vi "Assigning VICI Letter.vi"() -> ()   [LabVIEW 2018, in "VICI M6 M50 Party Mode.lvlib"]
uses:
  VICI M6 M50 Party Mode.lvlib
  <vilib>/Instr/_visa.llb/VISA Configure Serial Port (Instr).vi
panel:
  out "Bytes at Port 5":u32
  out "read buffer 8":string
  out "String 2":string
  out "Bytes at Port 7":u32
  out "read buffer 3":string
  out "Already Labeled":bool
  out "error out":errorcluster
  out "String":string
  out "Bytes at Port 6":u32
  out "read buffer 2":string
  out "output array":string[](array[string])
  out "Bytes at Port 4":u32
  out "read buffer 7":string
  out "Bytes at Port 3":u32
  out "read buffer 6":string
  in  "VISA resource name":refnum<visa-resource-name>
  in  "error in (no error)":errorcluster
  out "read buffer 5":string
  out "Bytes at Port":u32
  out "read buffer":string
  out "Bytes at Port 2":u32
  in  "Pump Letter (single, case sensitive letter of number)":string
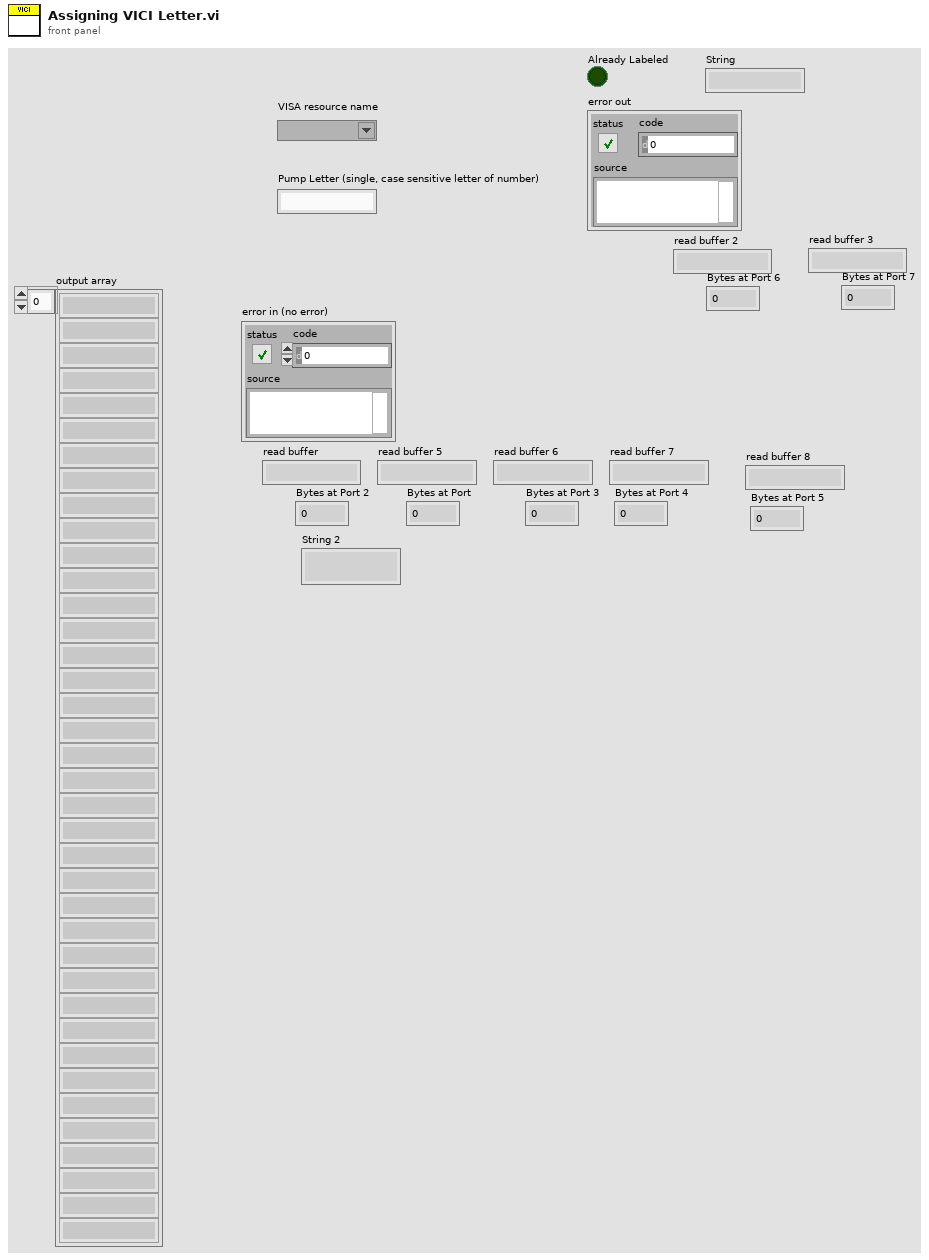
[diagram p1: front panel]
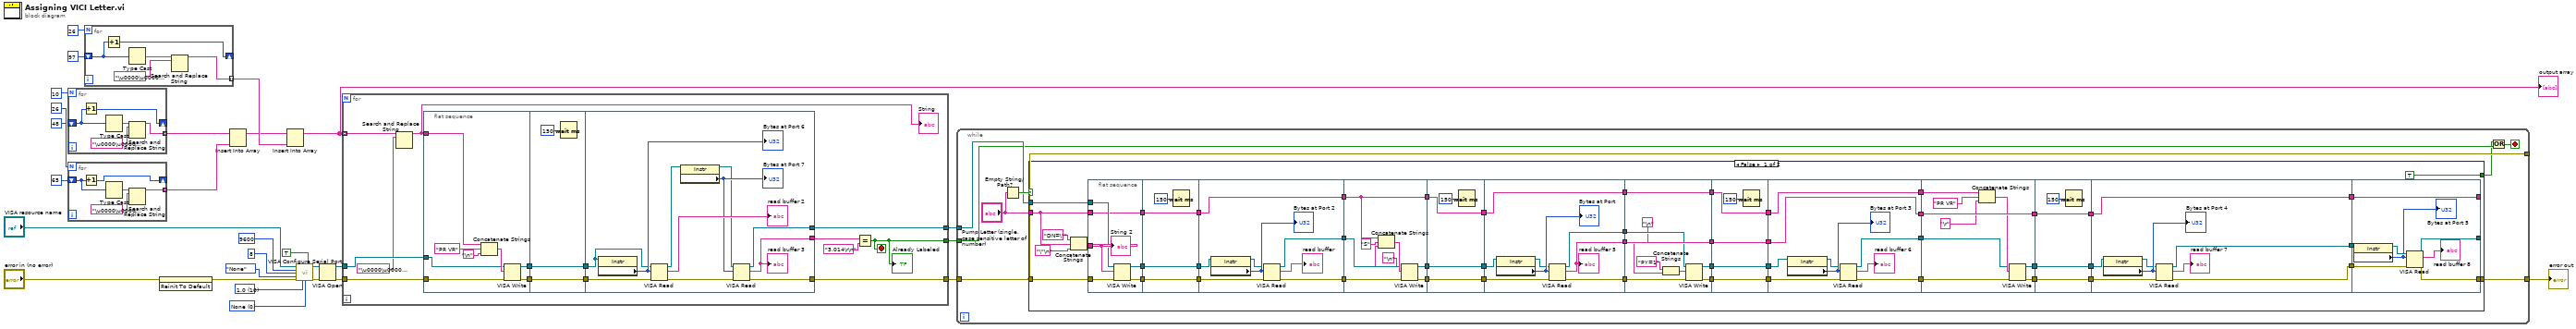
[diagram p0: block diagram]
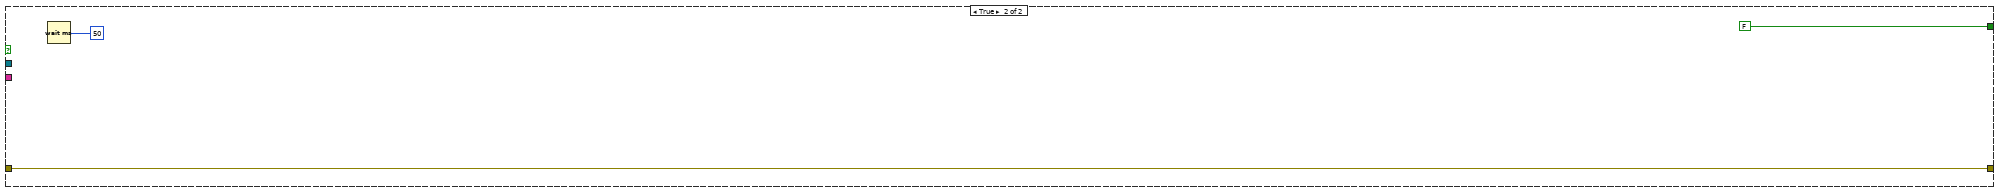
[diagram p2: hidden frame]
diagram:
  w23 = u16 0 items=["None", "XON/XOFF", "RTS/CTS", "XON/XOFF & RTS/CTS", "DTR/DSR", "XON/XOFF & DTR/DSR"] ("flow control (0:none)")
  w24 = u16 10 items=["1.0"=10, "1.5"=15, "2.0"=20] ("stop bits (10: 1 bit)")
  n1 = for {
    N: 10 -> [_]
    shift-right: [w33] -> _
    shift-left: 48 -> [w32]
    tunnel: [w29] -> w8 mode=indexing
    n2 = Increment(x=w32) -> (x+1=w33:i32)
    n3 = Type Cast(x=w32) -> (*(type *) &x=w30:string)  [unwired: 1 in]
    n4 = Search and Replace String(input string=w30, search string="\u0000\u0000\u0000") -> (result string=w29:string)  [unwired: 6 in, 3 out]
  }
  n5 = for {
    N: 26 -> [_]
    shift-right: [w38] -> _
    shift-left: 65 -> [w37]
    tunnel: [w34] -> w9 mode=indexing
    n6 = Increment(x=w37) -> (x+1=w38:i32)
    n7 = Type Cast(x=w37) -> (*(type *) &x=w35:string)  [unwired: 1 in]
    n8 = Search and Replace String(input string=w35, search string="\u0000\u0000\u0000") -> (result string=w34:string)  [unwired: 6 in, 3 out]
  }
  n9 = for {
    N: 26 -> [_]
    shift-right: [w43] -> _
    shift-left: 97 -> [w42]
    tunnel: [w39] -> w11 mode=indexing
    n10 = Increment(x=w42) -> (x+1=w43:i32)
    n11 = Type Cast(x=w42) -> (*(type *) &x=w40:string)  [unwired: 1 in]
    n12 = Search and Replace String(input string=w40, search string="\u0000\u0000\u0000") -> (result string=w39:string)  [unwired: 6 in, 3 out]
  }
  n13 = invoke on="Pump Letter (single, case sensitive letter of number)" class="Str" method="Reinit To Default"(error in="error in (no error)") -> (error out=w19:errorcluster)  [unwired: 2 in, 2 out]
  n14 = Insert Into Array(array=w8, new element=w9) -> (w10:string[])  [unwired: 1 in]
  n15 = Insert Into Array(array=w10, new element=w11) -> (w1:string[])  [unwired: 1 in]
  "output array" <- w1
  n16 = call-poly "VISA Configure Serial Port"("VISA resource name"="VISA resource name", "Enable Termination\nChar (T)"=TRUE ("Enable Termination\nChar (T)"), "baud rate (9600)"=u32 9600, "data bits (8)"=u16 8, "parity (0:none)"=enum16{"None", "Odd", "Even", "Mark", "Space"}."None", "error in (no error)"=w19, "stop bits (10: 1 bit)"=w24, "flow control (0:none)"=w23) -> ("VISA resource name out"=w21:refnum<visa-resource-name>, "error out"=w22:errorcluster)  [unwired: 6 in]
  n17 = VISA Open(error in (no error)=w22, VISA resource name=w21) -> (VISA resource name=w16:refnum<visa-resource-name>, error out=w17:errorcluster)  [unwired: 3 in]
  n18 = for {
    tunnel: w1 -> [w48] mode=indexing
    tunnel: w17 -> [w53]
    tunnel: w16 -> [w52]
    tunnel: [w50] -> w13
    tunnel: [w49] -> w14
    tunnel: [w44] -> w12
    stop <- w44 stop-if-true
    n19 = Search and Replace String(input string=w48, search string="\u0000\u0000\u0000") -> (result string=w47:string)  [unwired: 6 in, 3 out]
    "String" <- w47
    n20 = flat-sequence {
      tunnel: w47 -> [w64]
      tunnel: [w63] -> w56
      tunnel: [w62] -> w55
      tunnel: w53 -> [w61]
      tunnel: w52 -> [w60]
      tunnel: [w67] -> w57
      tunnel: w56 -> [w67]
      tunnel: w55 -> [w66]
      tunnel: [w66] -> w54
      tunnel: w57 -> [w78]
      tunnel: w54 -> [w77]
      tunnel: [w72] -> w50
      tunnel: [w74] -> w49
      tunnel: [w69] -> w45
      frame #0 {
        n21 = Concatenate Strings(w64, "PR VR" ("string"), "\n") -> (w65:string)
        n22 = VISA Write(VISA resource name=w60, write buffer=w65, error in (no error)=w61) -> (VISA resource name out=w63:refnum<visa-resource-name>, error out=w62:errorcluster)  [unwired: 1 out]
      }
      frame #1 {
        n23 = Wait (ms)(milliseconds to wait=u32 150) -> ()  [unwired: 1 out]
      }
      frame #2 {
        n24 = property class="Instr"(reference=w78) -> ("Serial Settings:Number of Bytes at Serial Port"=w79:u32)  [unwired: 1 in, 2 out]
        "Bytes at Port 6" <- w79
        n25 = VISA Read(VISA resource name=w78, byte count=w79, error in (no error)=w77) -> (VISA resource name out=w71:refnum<visa-resource-name>, read buffer=→"read buffer 2":string, error out=w73:errorcluster)  [unwired: 1 out]
        n26 = property class="Instr"(reference=w71) -> (reference out=w70:refnum<visa-resource-name>, "Serial Settings:Number of Bytes at Serial Port"=w75:u32)  [unwired: 1 in, 1 out]
        "Bytes at Port 7" <- w75
        n27 = VISA Read(VISA resource name=w70, byte count=w75, error in (no error)=w73) -> (VISA resource name out=w74:refnum<visa-resource-name>, read buffer=w69:string, error out=w72:errorcluster)  [unwired: 1 out]
        "read buffer 3" <- w69
      }
    }
    n28 = Equal?(x=w45, y="3.014\r\n") -> (x = y?=w44:bool)
    "Already Labeled" <- w44
  }
  n29 = while {
    tunnel: [w84] -> _
    tunnel: w14 -> [w85]
    tunnel: w13 -> [w84]
    tunnel: [w83] -> w15
    tunnel: w12 -> [w82]
    stop <- w80 stop-if-true
    n30 = Empty String/Path?(string/path="Pump Letter (single, case sensitive letter of number)") -> (empty?=w87:bool)
    n31 = case shown="False" w87 {
      tunnel: "Pump Letter (single, case sensitive letter of number)" -> [w117 _]
      tunnel: w84 -> [w122 w226]
      tunnel: [TRUE FALSE] -> w81
      tunnel: w85 -> [w121 _]
      tunnel: [w120 w226] -> w83
      frame False {
        n32 = Concatenate Strings("DN=\"" ("string"), w117, "\"\n" ("string")) -> (w116:string)
        n33 = flat-sequence {
          tunnel: [w140] -> w135
          tunnel: [w139] -> w134
          tunnel: w122 -> [w141]
          tunnel: w117 -> [w136]
          tunnel: w121 -> [w138]
          tunnel: w116 -> [w137]
          tunnel: [w136] -> w113
          tunnel: [w143] -> w133
          tunnel: w135 -> [w143]
          tunnel: w134 -> [w144]
          tunnel: [w144] -> w132
          tunnel: [w142] -> w114
          tunnel: w113 -> [w142]
          tunnel: w133 -> [w149]
          tunnel: w132 -> [w153]
          tunnel: [w151] -> w131
          tunnel: [w150] -> w130
          tunnel: [w147] -> w115
          tunnel: w114 -> [w147]
          tunnel: w131 -> [w157]
          tunnel: [w155] -> w110
          tunnel: w130 -> [w158]
          tunnel: [w156] -> w108
          tunnel: w115 -> [w159]
          tunnel: [w159] -> w106
          tunnel: w110 -> [w165]
          tunnel: [w165] -> w109
          tunnel: w108 -> [w164]
          tunnel: [w164] -> w107
          tunnel: w106 -> [w163]
          tunnel: [w163] -> w105
          tunnel: w109 -> [w173]
          tunnel: w107 -> [w169]
          tunnel: [w172] -> w128
          tunnel: [w171] -> w127
          tunnel: [w170] -> w126
          tunnel: w105 -> [w167]
          tunnel: [w167] -> w112
          tunnel: w128 -> [w177]
          tunnel: w127 -> [w182]
          tunnel: w126 -> [w179]
          tunnel: [w176] -> w104
          tunnel: [w182] -> w102
          tunnel: [w178] -> w100
          tunnel: w112 -> [w175]
          tunnel: [w175] -> w98
          tunnel: w104 -> [w187]
          tunnel: [w187] -> w103
          tunnel: w102 -> [w186]
          tunnel: [w186] -> w101
          tunnel: w100 -> [w185]
          tunnel: [w185] -> w99
          tunnel: w98 -> [w184]
          tunnel: [w184] -> w97
          tunnel: w103 -> [w191]
          tunnel: w101 -> [w196]
          tunnel: w99 -> [w193]
          tunnel: [w190] -> w125
          tunnel: [w196] -> w124
          tunnel: [w192] -> w123
          tunnel: w97 -> [w189]
          tunnel: [w189] -> w111
          tunnel: w125 -> [w200]
          tunnel: w124 -> [w205]
          tunnel: w123 -> [w201]
          tunnel: [w198] -> w96
          tunnel: [w205] -> w94
          tunnel: [w199] -> w92
          tunnel: w111 -> [w202]
          tunnel: w96 -> [w209]
          tunnel: [w209] -> w95
          tunnel: w94 -> [w208]
          tunnel: [w208] -> w93
          tunnel: w92 -> [w207]
          tunnel: [w207] -> w91
          tunnel: w95 -> [w213]
          tunnel: w93 -> [w217]
          tunnel: w91 -> [w214]
          tunnel: [w217] -> w90
          tunnel: [w211] -> w89
          tunnel: [w210] -> w88
          tunnel: [w218] -> _
          tunnel: [w225] -> _
          tunnel: [w219] -> w120
          tunnel: w90 -> [w225]
          tunnel: w89 -> [w221]
          tunnel: w88 -> [w220]
          frame #0 {
            n34 = VISA Write(VISA resource name=w138, write buffer=w137, error in (no error)=w141) -> (VISA resource name out=w140:refnum<visa-resource-name>, error out=w139:errorcluster)  [unwired: 1 out]
            "String 2" <- w137
          }
          frame #1 {
            n35 = Wait (ms)(milliseconds to wait=u32 150) -> ()  [unwired: 1 out]
          }
          frame #2 {
            n36 = property class="Instr"(reference=w149) -> (reference out=w146:refnum<visa-resource-name>, "Serial Settings:Number of Bytes at Serial Port"=w148:u32)  [unwired: 1 in, 1 out]
            "Bytes at Port 2" <- w148
            n37 = VISA Read(VISA resource name=w146, byte count=w148, error in (no error)=w153) -> (VISA resource name out=w150:refnum<visa-resource-name>, read buffer=→"read buffer":string, error out=w151:errorcluster)  [unwired: 1 out]
          }
          frame #3 {
            n38 = Concatenate Strings(w159, "S" ("string"), "\n" ("string")) -> (w160:string)
            n39 = VISA Write(VISA resource name=w158, write buffer=w160, error in (no error)=w157) -> (VISA resource name out=w156:refnum<visa-resource-name>, error out=w155:errorcluster)  [unwired: 1 out]
          }
          frame #4 {
            n40 = Wait (ms)(milliseconds to wait=u32 150) -> ()  [unwired: 1 out]
          }
          frame #5 {
            n41 = property class="Instr"(reference=w169) -> (reference out=w166:refnum<visa-resource-name>, "Serial Settings:Number of Bytes at Serial Port"=w168:u32)  [unwired: 1 in, 1 out]
            "Bytes at Port" <- w168
            n42 = VISA Read(VISA resource name=w166, byte count=w168, error in (no error)=w173) -> (VISA resource name out=w170:refnum<visa-resource-name>, read buffer=w171:string, error out=w172:errorcluster)  [unwired: 1 out]
            "read buffer 5" <- w171
          }
          frame #6 {
            n43 = Concatenate Strings("PY=1" ("string"), "\n" ("string")) -> (w180:string)
            n44 = VISA Write(VISA resource name=w179, write buffer=w180, error in (no error)=w177) -> (VISA resource name out=w178:refnum<visa-resource-name>, error out=w176:errorcluster)  [unwired: 1 out]
          }
          frame #7 {
            n45 = Wait (ms)(milliseconds to wait=u32 150) -> ()  [unwired: 1 out]
          }
          frame #8 {
            n46 = property class="Instr"(reference=w193) -> (reference out=w188:refnum<visa-resource-name>, "Serial Settings:Number of Bytes at Serial Port"=w194:u32)  [unwired: 1 in, 1 out]
            "Bytes at Port 3" <- w194
            n47 = VISA Read(VISA resource name=w188, byte count=w194, error in (no error)=w191) -> (VISA resource name out=w192:refnum<visa-resource-name>, read buffer=→"read buffer 6":string, error out=w190:errorcluster)  [unwired: 1 out]
          }
          frame #9 {
            n48 = Concatenate Strings(w202, "PR VR" ("string"), "\r" ("string")) -> (w203:string)
            n49 = VISA Write(VISA resource name=w201, write buffer=w203, error in (no error)=w200) -> (VISA resource name out=w199:refnum<visa-resource-name>, error out=w198:errorcluster)  [unwired: 1 out]
          }
          frame #10 {
            n50 = Wait (ms)(milliseconds to wait=u32 150) -> ()  [unwired: 1 out]
          }
          frame #11 {
            n51 = property class="Instr"(reference=w214) -> (reference out=w212:refnum<visa-resource-name>, "Serial Settings:Number of Bytes at Serial Port"=w215:u32)  [unwired: 1 in, 1 out]
            "Bytes at Port 4" <- w215
            n52 = VISA Read(VISA resource name=w212, byte count=w215, error in (no error)=w213) -> (VISA resource name out=w211:refnum<visa-resource-name>, read buffer=→"read buffer 7":string, error out=w210:errorcluster)  [unwired: 1 out]
          }
          frame #12 {
            n53 = property class="Instr"(reference=w221) -> (reference out=w224:refnum<visa-resource-name>, "Serial Settings:Number of Bytes at Serial Port"=w223:u32)  [unwired: 1 in, 1 out]
            "Bytes at Port 5" <- w223
            n54 = VISA Read(VISA resource name=w224, byte count=w223, error in (no error)=w220) -> (VISA resource name out=w218:refnum<visa-resource-name>, read buffer=→"read buffer 8":string, error out=w219:errorcluster)  [unwired: 1 out]
          }
        }
      }
      frame True {
        n55 = Wait (ms)(milliseconds to wait=u32 50) -> ()  [unwired: 1 out]
      }
    }
    n56 = Or(x=w81, y=w82) -> (x .or. y?=w80:bool)
  }
  "error out" <- w15
